vi "Build Preview.vi"(6 "Average During Loop ?":bool, 8 "error in (no error)":errorcluster, 9 "Loop ?":cluster{i32, i32}, 10 "Program":T1(array[cluster]), 11 "# Of Loops":u32) -> (0 "error out":errorcluster, 1 "Measure ? Out":bool[](array[boolean]), 2 "Y Values Out":dbl[](array[numeric]), 3 "Storage Locations Out":i32[](array[numeric]), 4 "Direction Out":bool[](array[boolean]), 5 "Plots Out":cluster{dbl[], dbl[]}[](array[cluster]), 7 "Stage Values":i32[](array[numeric]))   [LabVIEW 2012, in "Multi Segment Waveform.xctl"]
doc: "Builds a set of X-Y plots based on the current program and loop settings ."
uses:
  Multi Segment Waveform.xctl
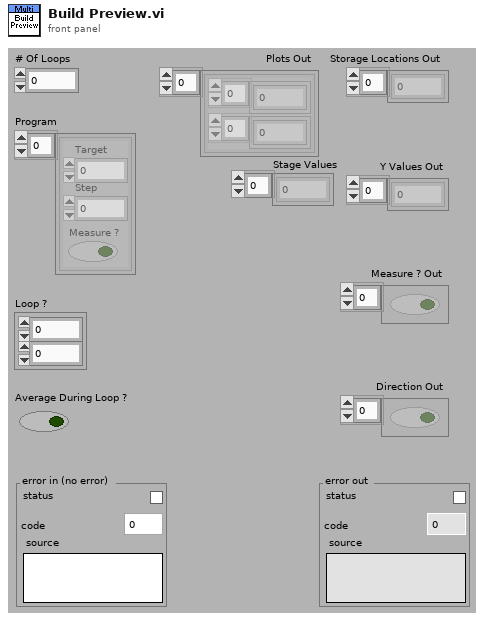
[diagram p1: front panel]
types:
  T1 = cluster{"Target":dbl, "Step":dbl, "Measure ?":bool}[]
  T2 = cluster{"Storage Locs":i32[], "Measure":bool[], "Field":dbl[], "Direction":bool[]}
  T3 = cluster{"Target":dbl, "Step":dbl, "Measure ?":bool}
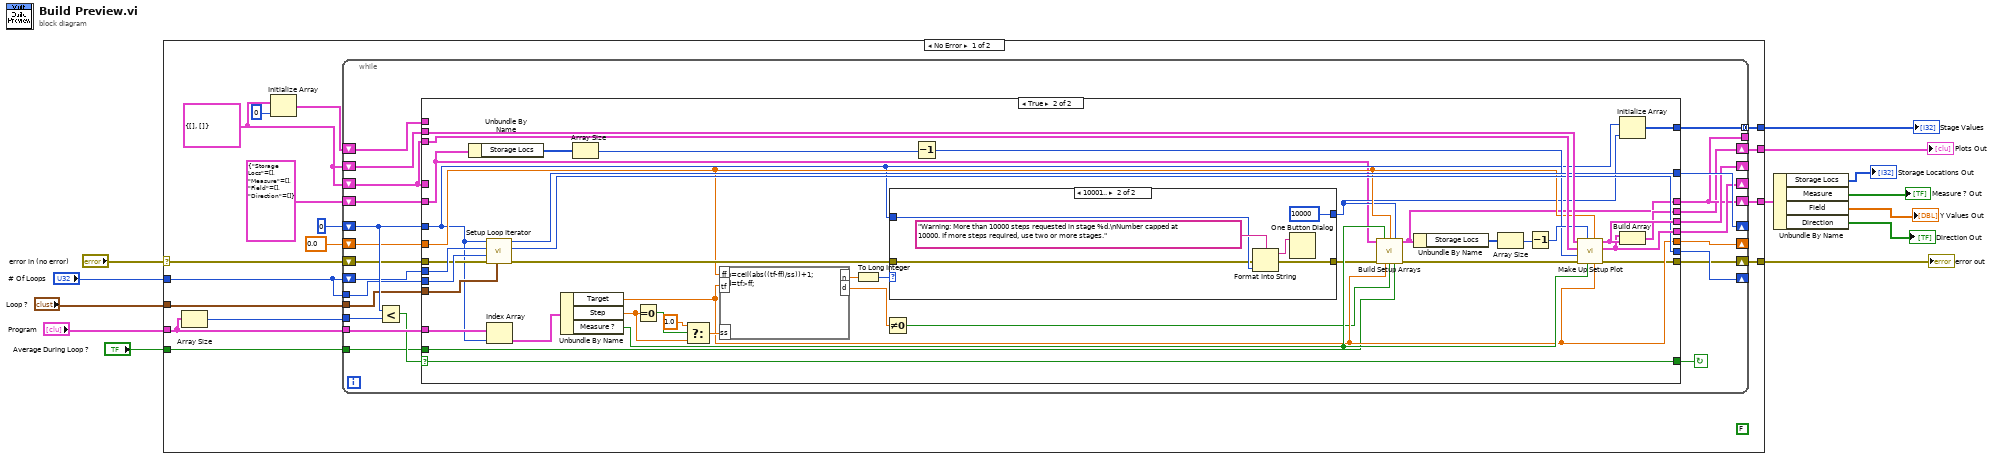
[diagram p0: block diagram]
diagram:
  n1 = case shown="No Error" "error in (no error)" {
    selector: "error in (no error)" -> [w17 w112]
    tunnel: [w26 _] -> w13
    tunnel: "Average During Loop ?" -> [w25 _]
    tunnel: "Loop ?" -> [w24 _]
    tunnel: "Program" -> [w23 _]
    tunnel: "# Of Loops" -> [w19 _]
    tunnel: [w18 _] -> w5
    tunnel: [w16 w112] -> w7
    tunnel: [w15 _] -> w6
    frame No Error {
      w27 = cluster{dbl[], dbl[]} {[], []}
      (unwired) FALSE
      n2 = Array Size(array=w23) -> (size(s)=w21:i32)
      n3 = Initialize Array(w27, 0 ("dimension size")) -> (w28:cluster{dbl[], dbl[]}[])
      n4 = while {
        tunnel: [w37] -> _
        shift-left: T2 {"Storage Locs"=[], "Measure"=[], "Field"=[], "Direction"=[]} ("Preview Out") -> [w38]
        shift-right: [w37] -> w18
        tunnel: w19 -> [w39]
        shift-left: w27 -> [w43]
        shift-right: [w42] -> _
        shift-left: w27 -> [w40]
        shift-right: [w41] -> _
        shift-left: w19 -> [w48]
        shift-right: [w47] -> _
        tunnel: w21 -> [w51]
        shift-left: 0 -> [w53]
        shift-right: [w46] -> _
        shift-left: 0.0 -> [w45]
        shift-right: [w44] -> _
        tunnel: w23 -> [w52]
        tunnel: w24 -> [w36]
        tunnel: w25 -> [w34]
        shift-right: [w35] -> w26
        shift-left: w28 -> [w33]
        shift-right: [w32] -> w16
        shift-left: w17 -> [w31]
        tunnel: [w30] -> w15 mode=concatenating
        stop <- w49 continue-if-true
        n5 = Less?(x=w53, y=w51) -> (x < y?=w50:bool)
        n6 = case shown="True" w50 {
          selector: w50 -> [w62 w93]
          tunnel: w53 -> [w60 w68]
          tunnel: w52 -> [_ w103]
          tunnel: [w62 w93] -> w49
          tunnel: w48 -> [w61 w96]
          tunnel: [w61 w95] -> w47
          tunnel: [w60 w94] -> w46
          tunnel: w45 -> [w59 w74]
          tunnel: [w59 w79] -> w44
          tunnel: w40 -> [_ w99]
          tunnel: w43 -> [w57 w98]
          tunnel: [w57 w101] -> w42
          tunnel: [w58 w100] -> w41
          tunnel: w40 -> [w58 _]
          tunnel: w39 -> [_ w97]
          tunnel: w38 -> [w56 w66]
          tunnel: [w56 w64] -> w37
          tunnel: w36 -> [_ w78]
          tunnel: [w55 w85] -> w35
          tunnel: w34 -> [_ w72]
          tunnel: w33 -> [w55 _]
          tunnel: [w54 w70] -> w32
          tunnel: w31 -> [w54 w77]
          tunnel: [_ w67] -> w30
          frame False {
          }
          frame True {
            n7 = Unbundle By Name(w66) -> ("Storage Locs"=w65:i32[])
            n8 = call "Setup Loop Iterator.vi"("Loop"=w78, "error in (no error)"=w77, "Total Loops"=w97, "Loop Iterator"=w96, "Previous Line"=w68) -> ("error out"=w76:errorcluster, "Loop Iterator Out"=w95:u32, "Line Iterator Out"=w94:i32)  [unwired: 4 out]
            n9 = Index Array(array=w103, index=w68) -> (element=w102:T3)
            n10 = Unbundle By Name(w102) -> ("Target"=w79:dbl, "Step"=w82:dbl, "Measure ?"=w86:bool)
            n11 = Array Size(array=w65) -> (size(s)=w88:i32)
            n12 = Equal To 0?(x=w82) -> (x = 0?=w84:bool)
            n13 = Select(t=1.0, s=w84, f=w82) -> (s? t:f=w81:dbl)
            n14 = formula code="n=ceil(abs((tf-ff)/ss))+1;\nd=tf>ff;"("ff"=w74, "tf"=w79, "ss"=w81) -> ("n"=w91:dbl, "d"=w92:dbl)
            n15 = To Long Integer(number=w91) -> (32bit integer=w80:i32)
            n16 = Not Equal To 0?(x=w92) -> (x != 0?=w73:bool)
            n17 = case shown="10001.." w80 {
              selector: w80 -> [w105 _]
              tunnel: [w105 10000] -> w69
              tunnel: w68 -> [_ w109]
              tunnel: w76 -> [w104 w107]
              tunnel: [w104 w106] -> w75
              frame ..10000 {
              }
              frame 10001.. {
                n18 = Format Into String(format string="Warning: More than 10000 steps requested in stage %d.\nNumber capped at 10000. If more steps required, use two or more stages.", error in=w107, w109) -> (resulting string=w108:string, error out=w106:errorcluster)  [unwired: 1 in]
                n19 = One Button Dialog(message=w108) -> ()  [unwired: 2 out]
              }
            }
            n20 = Decrement(x=w88) -> (x-1=w87:i32)
            n21 = call "Build Setup Arrays.vi"("Preview In"=w66, "Measure ?"=w86, "First Field"=w74, "N Points"=w69, "error in (no error)"=w75, "Last Field"=w79, "Direction"=w73, "Average During Loop ?"=w72) -> ("Preview Out"=w64:T2, "error out"=w71:errorcluster)  [unwired: 3 in, 3 out]
            n22 = Unbundle By Name(w64) -> ("Storage Locs"=w63:i32[])
            n23 = Array Size(array=w63) -> (size(s)=w90:i32)
            n24 = Decrement(x=w90) -> (x-1=w89:i32)
            n25 = call "Make Up Setup Plot.vi"("End Field"=w79, "Start Field"=w74, "Put in plot 1"=w86, "End X"=w89, "error in (no error)"=w71, "Start X"=w87, "Plot 1 In"=w99, "Plot 2 In"=w98) -> ("error out"=w70:errorcluster, "Plot 1 Out"=w100:cluster{dbl[], dbl[]}, "Plot 2 Out"=w101:cluster{dbl[], dbl[]})  [unwired: 1 out]
            n26 = Initialize Array(w68, w69) -> (w67:i32[])
            n27 = Build Array(w100, w101) -> (w85:cluster{dbl[], dbl[]}[])
          }
        }
      }
    }
    frame Error {
    }
  }
  "Plots Out" <- w13
  "error out" <- w7
  "Stage Values" <- w6
  n28 = Unbundle By Name(w5) -> ("Storage Locs"=→"Storage Locations Out":i32[], "Measure"=→"Measure ? Out":bool[], "Field"=→"Y Values Out":dbl[], "Direction"=→"Direction Out":bool[])
